vi "processData.vi"(8 "error in (no error)":errorcluster, 10 "model":refnum<class "Model.lvclass">, 11 "PausingState in":refnum<class "PausingState.lvclass">) -> (0 "error out":errorcluster, 2 "model 2":refnum<class "Model.lvclass">, 3 "PausingState out":refnum<class "PausingState.lvclass">)   [LabVIEW 2013, in "PausingState.lvclass"]
uses:
  PausingState.lvclass
  Model/Model/Model.lvclass
  ExecutingCycleState/ExecutingCycleState.lvclass
  Typedefs/StateSelector.ctl
  Typedefs/M2AADTTypedefs.lvlib
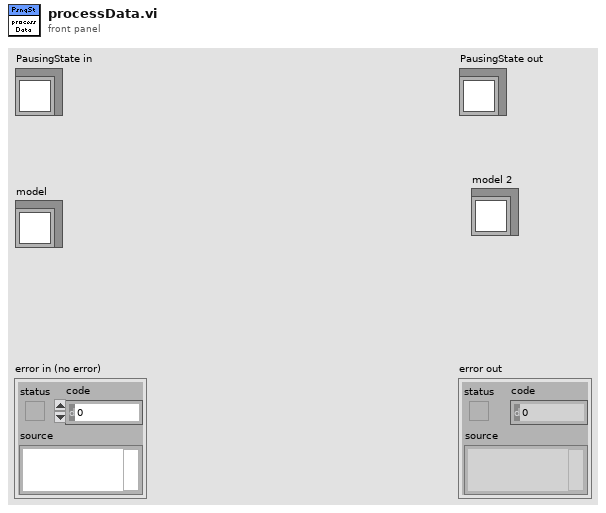
[diagram p1: front panel]
types:
  T1 = typedef "M2AADTTypedefs.lvlib/StateSelector.ctl" = enum16{"EndingCycleState", "FaultState", "InteractiveMotionState", "MovingToNewForceState", "OffState", "PausingState", "StandbyState", "StoppedState"}
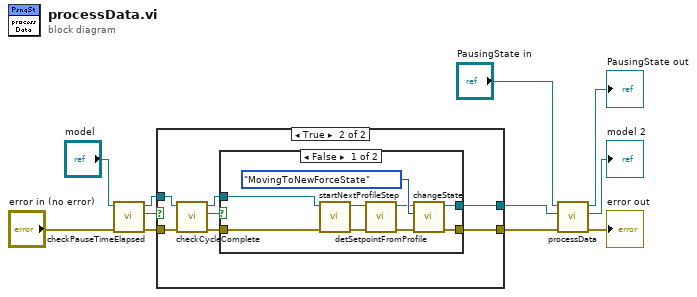
[diagram p0: block diagram]
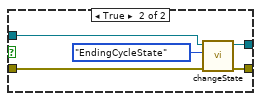
[diagram p3: hidden frame]
diagram:
  n1 = call "checkPauseTimeElapsed.vi"("error in (no error)"="error in (no error)", "Model in"="model") -> ("error out"=w2:errorcluster, "pauseTimeHasElapsedIsTrue"=w7:bool, "Model out"=w5:refnum<class "Model.lvclass">)  [unwired: 7 in]
  n2 = case shown="True" w7 {
    tunnel: w5 -> [w13 w20]
    tunnel: [w13 w18] -> w4
    tunnel: w2 -> [w12 w17]
    tunnel: [w12 w14] -> w1
    frame False {
    }
    frame True {
      n3 = call "checkCycleComplete.vi"("error in (no error)"=w17, "Model in"=w20) -> ("error out"=w16:errorcluster, "cycleCompleteIsTrue"=w15:bool, "Model out"=w19:refnum<class "Model.lvclass">)  [unwired: 7 in]
      n4 = case shown="False" w15 {
        tunnel: w19 -> [w28 w33]
        tunnel: [w27 w32] -> w18
        tunnel: w16 -> [w26 w31]
        tunnel: [w25 w30] -> w14
        frame False {
          n5 = call "startNextProfileStep.vi"("error in (no error)"=w26, "Model in"=w28) -> ("error out"=w22:errorcluster, "Model out"=w24:refnum<class "Model.lvclass">)  [unwired: 8 in]
          n6 = call "detSetpointFromProfile.vi"("error in (no error)"=w22, "Model in"=w24) -> ("error out"=w21:errorcluster, "Model out"=w23:refnum<class "Model.lvclass">)  [unwired: 8 in]
          n7 = call "changeState.vi"("error in (no error)"=w21, "State:"=StateSelector."MovingToNewForceState", "Model in"=w23) -> ("error out"=w25:errorcluster, "Model out"=w27:refnum<class "Model.lvclass">)  [unwired: 7 in]
        }
        frame True {
          n8 = call "changeState.vi"("error in (no error)"=w31, "State:"=StateSelector."EndingCycleState", "Model in"=w33) -> ("error out"=w30:errorcluster, "Model out"=w32:refnum<class "Model.lvclass">)  [unwired: 7 in]
        }
      }
    }
  }
  n9 = call-parent "processData.vi"("error in (no error)"=w1, "model"=w4, "ControlledMotionState in"="PausingState in") -> ("error out"=→"error out":errorcluster, "model 2"=→"model 2":refnum<class "Model.lvclass">, "ControlledMotionState out"=→"PausingState out":refnum<class "PausingState.lvclass">)  [unwired: 6 in]
